vi "4bloginpage.vi"() -> ()   [LabVIEW 2013]
panel:
  out "Success":bool
  in  "Login Page":T1
  # "4b) Login page creation using cluster\n23A91A0459\nS.NIKHIL PRINCE"
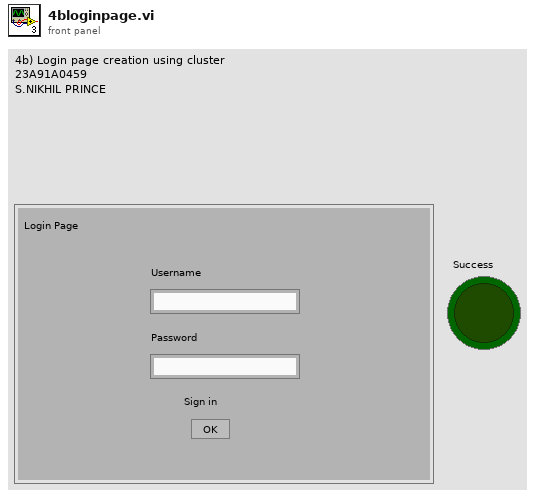
[diagram p1: front panel]
types:
  T1 = cluster{"Username":string, "Password":string, "Sign in":bool}
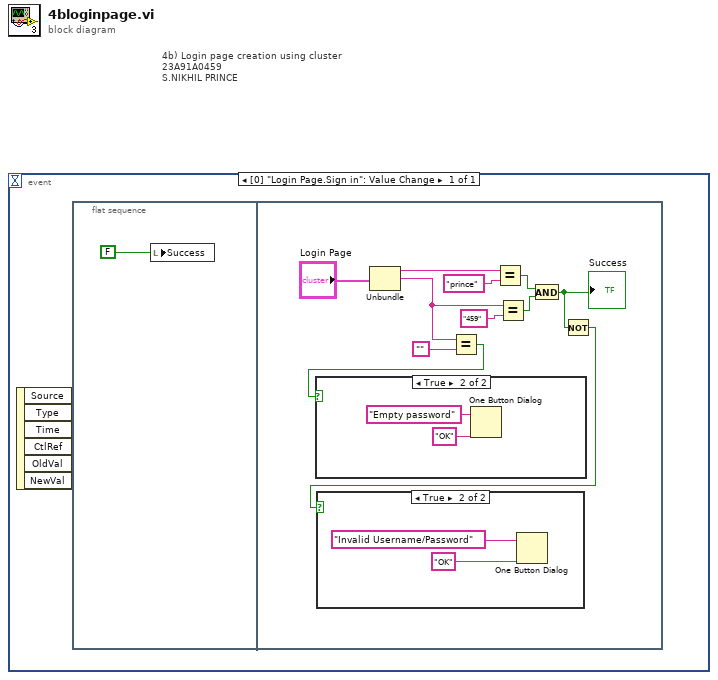
[diagram p0: block diagram]
diagram:
  # "4b) Login page creation using cluster\n23A91A0459\nS.NIKHIL PRINCE"
  n1 = event shown="[0] \"Login Page.Sign in\": Value Change" {
    selector: _ -> [_]
    dyn-events: _ -> [_]
    timeout: _ -> [_]
    event "Login Page.Sign in": Value Change {
      n2 = event-data() -> ()  [unwired: 1 in, 6 out]
      n3 = flat-sequence {
        frame #0 {
          n4 = local write "Success"(FALSE) -> ()
        }
        frame #1 {
          n5 = Unbundle "Unbundle"("Login Page") -> ("Username"=w11:string, "Password"=w6:string)  [unwired: 1 out]
          n6 = Equal?(x=w6, y="") -> (x = y?=w5:bool)
          n7 = case shown="True" w5 {
            frame False {
            }
            frame True {
              n8 = One Button Dialog(message="Empty password", button name ("OK")="OK") -> ()  [unwired: 1 out]
            }
          }
          n9 = Equal?(x=w11, y="prince") -> (x = y?=w8:bool)
          n10 = Equal?(x=w6, y="459") -> (x = y?=w7:bool)
          n11 = And(x=w8, y=w7) -> (x .and. y?=w3:bool)
          "Success" <- w3
          n12 = Not(x=w3) -> (.not. x?=w2:bool)
          n13 = case shown="True" w2 {
            frame False {
            }
            frame True {
              n14 = One Button Dialog(message="Invalid Username/Password", button name ("OK")="OK") -> ()  [unwired: 1 out]
            }
          }
        }
      }
    }
  }
